vi "Perform Measurement.vi"(7 "error in (no error)":errorcluster, 8 "Measure Call Context in":refnum<class "Measure Call Context.lvclass">, 10 "measurement configuration":T2={"Mode of operation"=enum."Power on the DUT", "Source enable/disable"=FALSE, "Load enable/disable"=FALSE, "Source resource names"=[], "Load resource names"=[], "Power ON/Source system configuration"=enum."Series", "Power ON/Source output function"=0, "Source sweep scale"="", "Power ON V/I Source start level"=0.0, "Source stop level"=0.0, "Source sweep points/points per decade"=0, "Source voltage/current level range"=0.0, "Power ON/Source sense"=0, "Source limit symmetry"=enum."Symmetric", "Power ON/Source current/voltage limit range"=0.0, "Source current/voltage limit low"=0.0, "Source current/voltage limit high"=0.0, "Source source delay"=0.0, "Source aperture time"=0.0, "Source transient response"=0, "Source voltage/current gain bandwidth"=0.0, "Source voltage/current compensation frequency"=0.0, "Source voltage/current pole-zero ratio"=0.0, "Load system configuration"=enum."Series", "Load output function"=0, "Load device voltage/current rating"=50.0, "Load sweep scale"="", "Load start level"=0.0, "Load stop level"=0.0, "Load sweep points/points per decade"=0, "Load voltage/current level range"=0.0, "Load sense"=0, "Load limit symmetry"=enum."Symmetric", "Load current/voltage limit range"=0.0, "Load current/voltage limit low"=0.0, "Load current/voltage limit high"=0.0, "Load source delay"=0.0, "Load aperture time"=0.0, "Load transient response"=0, "Load voltage/current gain bandwidth"=0.0, "Load voltage/current compensation frequency"=0.0, "Load voltage/current pole-zero ratio"=0.0, "Load source trigger"="", "Load measure trigger"="", "Measurement timeout"=10.0} {"Measurement timeout" format="%.3p"; "Load device voltage/current rating" format="%#_6pA"; "Load output function" items=["DC Voltage"=1006, "DC Current"=1007, "Pulse Voltage"=1049, "Pulse Current"=1050]; "Power ON/Source output function" items=["DC Voltage"=1006, "DC Current"=1007, "Pulse Voltage"=1049, "Pulse Current"=1050]; "Load sweep points/points per decade" format="%#_6p"; "Power ON V/I Source start level" format="%#_6p"; "Load sense" items=["Symmetric", "Asymmetric"]; "Load transient response" items=["Slow"=1041, "Normal"=1038, "Fast"=1039, "Custom"=1042]; "Power ON/Source sense" items=["Local"=1008, "Remote"=1009]; "Source transient response" items=["Slow"=1041, "Normal"=1038, "Fast"=1039, "Custom"=1042]; "Load current/voltage limit low" format="%#_6p"; "Load current/voltage limit range" format="%#_6p"; "Load voltage/current level range" format="%#_6p"; "Source current/voltage limit high" format="%#_6p"; "Source current/voltage limit low" format="%#_6p"; "Power ON/Source current/voltage limit range" format="%#_6p"; "Source voltage/current level range" format="%#_6p"}) -> (0 "error out":errorcluster, 1 "Measure Call Context out":refnum<class "Measure Call Context.lvclass">, 3 "Measurement Results":T1)   [LabVIEW 2021, in "Sweep_Channel Ganging.lvlib"]
doc: "This VI Perform different API calls to do Sweep Measurement in different configurations of Source and Load like \n\nSingle-Ganged \nGanged-Ganged\nGanged-Single\nSingle-Single"
uses:
  Sweep_Channel Ganging.lvlib
  <vilib>/Plug-In SDKs/Measurements/Measure Call Context/Measure Call Context.lvclass
  Measurement Configuration.ctl
  Measurement Results.ctl
  Controls/Sweep perform meaasurement.ctl
  shared subVIs/ctl/NIDCPower_channel_ganging - ctl - ganged session.ctl
  shared subVIs/ctl/NIDCPower_channel_ganging - ctl - ganged config.ctl
  shared subVIs/ctl/NIDCPower_channel_ganging - ctl - channel mode.ctl
  shared/Single/controls/Initialize Resource Config-Single.ctl
  shared/Ganging/controls/Initialize Resource Config-Ganging.ctl
  shared/Single/controls/Source to Sequence Config-Single.ctl
  shared/Ganging/controls/Source to Sequence Config-Ganging.ctl
  shared/Single/controls/Load to Sequence Config-Single.ctl
  shared/Ganging/controls/Load to Sequence Config-Ganging.ctl
  <instrlib>/niDCPower/nidcpower.llb/niDCPower Wait For Event - Event.ctl
  shared/Common/controls/Start and Wait for Event.ctl
  Controls/Sweep fetch measurement control.ctl
  shared/Ganging/controls/Abort Single Point-Ganging.ctl
  shared/Single/controls/Abort Single Point-Single.ctl
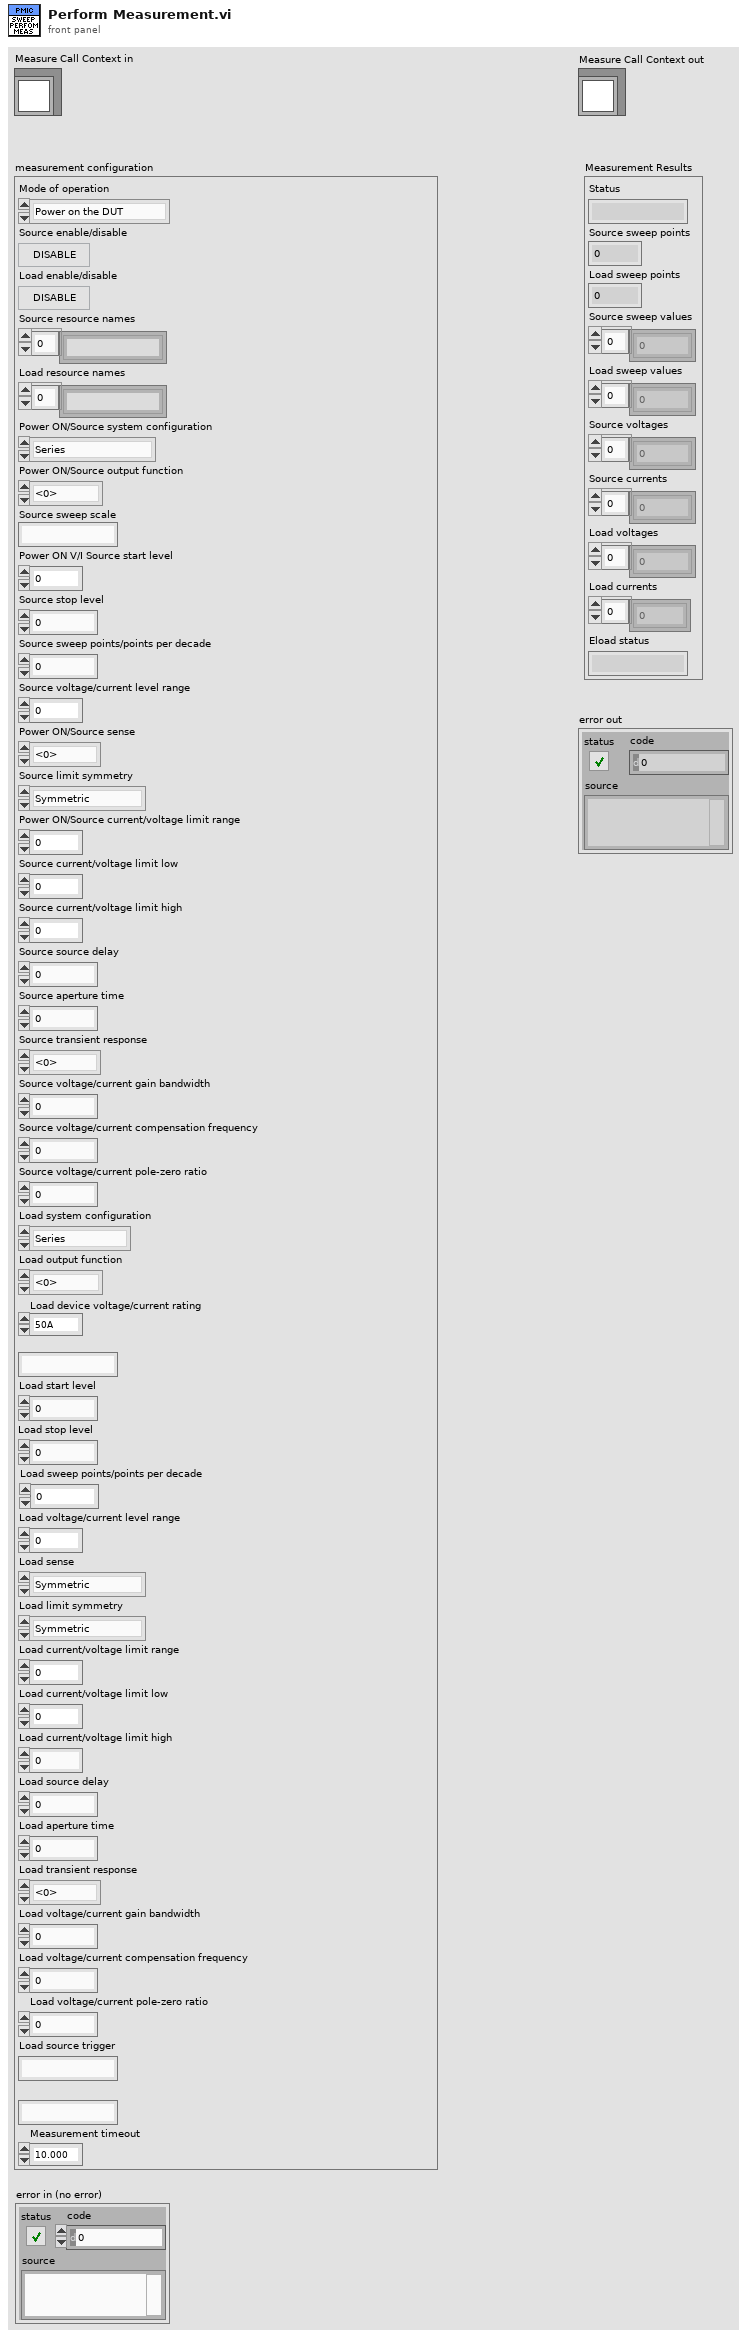
[diagram p1: front panel]
types:
  T1 = typedef "Sweep_Channel Ganging.lvlib/Measurement Results.ctl" = cluster{"Status":string, "Source sweep points":i32, "Load sweep points":i32, "Source sweep values":dbl[], "Load sweep values":dbl[], "Source voltages":dbl[], "Source currents":dbl[], "Load voltages":dbl[], "Load currents":dbl[], "Eload status":string}
  T2 = typedef "Sweep_Channel Ganging.lvlib/Measurement Configuration.ctl" = cluster{"Mode of operation":enum32{"Power on the DUT", "Perform measurement", "Power off the DUT"}, "Source enable/disable":bool, "Load enable/disable":bool, "Source resource names":string[], "Load resource names":string[], "Power ON/Source system configuration":enum32{"Series", "Parallel", "Manual"}, "Power ON/Source output function":i32, "Source sweep scale":string, "Power ON V/I Source start level":dbl, "Source stop level":dbl, "Source sweep points/points per decade":i32, "Source voltage/current level range":dbl, "Power ON/Source sense":i32, "Source limit symmetry":enum32{"Symmetric", "Asymmetric"}, "Power ON/Source current/voltage limit range":dbl, "Source current/voltage limit low":dbl, "Source current/voltage limit high":dbl, "Source source delay":dbl, "Source aperture time":dbl, "Source transient response":i32, "Source voltage/current gain bandwidth":dbl, "Source voltage/current compensation frequency":dbl, "Source voltage/current pole-zero ratio":dbl, "Load system configuration":enum32{"Series", "Parallel", "Manual"}, "Load output function":i32, "Load device voltage/current rating":dbl, "Load sweep scale":string, "Load start level":dbl, "Load stop level":dbl, "Load sweep points/points per decade":i32, "Load voltage/current level range":dbl, "Load sense":i32, "Load limit symmetry":enum32{"Symmetric", "Asymmetric"}, "Load current/voltage limit range":dbl, "Load current/voltage limit low":dbl, "Load current/voltage limit high":dbl, "Load source delay":dbl, "Load aperture time":dbl, "Load transient response":i32, "Load voltage/current gain bandwidth":dbl, "Load voltage/current compensation frequency":dbl, "Load voltage/current pole-zero ratio":dbl, "Load source trigger":string, "Load measure trigger":string, "Measurement timeout":dbl}
  T3 = typedef "Sweep_Channel Ganging.lvlib/Sweep perform meaasurement.ctl" = cluster{"Source Ganged Session Out":T4, "Load Ganged Session Out":T4, "Source sweep values":dbl[], "Source sweep points":i32, "Load sweep values":dbl[], "Load sweep points":i32, "Measurement Results":T1, "Source Master/Single resource name":string, "Source Slave resource name":string[], "Load Master/Single resource name":string, "Load Slave resource name":string[], "Load ganged/single":bool, "Source ganged/single":bool, "Source channel name":string, "Load channel name":string, "Source session out":refnum<k15>, "Load session out":refnum<k15>, "Number of Eload used":i32, "Load Source ON/OFF":enum16{"SOURCE AND LOAD OFF", "SOURCE ON", "LOAD ON", "SOURCE AND LOAD ON"}}
  T4 = typedef "NIDCPower_channel_ganging - ctl - ganged session.ctl" = cluster{"Ganged Config":T5, "Session List":refnum<k15>[], "Session Mode":T6[], "Channel":string[]}
  T5 = typedef "NIDCPower_channel_ganging - ctl - ganged config.ctl" = enum32{"Series", "Parallel", "Manual"}
  T6 = typedef "NIDCPower_channel_ganging - ctl - channel mode.ctl" = enum32{"Master", "Slave", "Slave - Inverted"}
  T7 = typedef "Initialize Resource Config-Single.ctl" = cluster{"Resource name":string, "Voltage/current level":dbl, "Voltage/current level range":dbl, "Voltage/current limit range":dbl, "Voltage/current limit low":dbl, "Voltage/current limit high":dbl, "Output function":i32, "Sense":i32, "Transient response":i32, "Voltage/current gain bandwidth":dbl, "Voltage/current compensation frequency":dbl, "Voltage/current pole-zero ratio":dbl, "DUT set-up time":dbl, "Limit symmetry":enum32{"Symmetric", "Asymmetric"}}
  T8 = typedef "Initialize Resource Config-Ganging.ctl" = cluster{"Master resource name ":string, "Slave resource names":string[], "System configuration":enum32{"Series", "Parallel", "Manual"}, "Voltage/current level":dbl, "Voltage/current level range":dbl, "Limit symmetry":enum32{"Symmetric", "Asymmetric"}, "Voltage/current limit range":dbl, "Voltage/current limit low":dbl, "Voltage/current limit high":dbl, "Output function":i32, "Sense":i32, "Transient response":i32, "Voltage/current gain bandwith":dbl, "Voltage/current compensation frequency":dbl, "Voltage/current pole-zero ratio":dbl, "DUT set-up time":dbl}
  T9 = typedef "Source to Sequence Config-Single.ctl" = cluster{"Source channel name":string, "Source out":refnum<k15>, "Source sweep values":dbl[], "Load sweep points":i32, "Source output function":i32, "Source transient response":i32, "Source voltage/current gain bandwidth":dbl, "Source voltage/current compensation frequency":dbl, "Source voltage/current pole-zero ratio":dbl, "Source aperture time":dbl, "Source source delay":dbl}
  T10 = typedef "Source to Sequence Config-Ganging.ctl" = cluster{"Source Ganged Session Out":cluster{"Ganged Config":T5, "Session List":refnum<k15>[], "Session Mode":T6[], "Channel":string[]}, "Source sweep values":dbl[], "Load sweep points":i32, "Source output function":i32, "Source transient response":i32, "Source voltage/current gain bandwidth":dbl, "Source voltage/current compensation frequency":dbl, "Source voltage/current pole-zero ratio":dbl, "Source aperture time":dbl, "Source source delay":dbl}
  T11 = typedef "Load to Sequence Config-Single.ctl" = cluster{"Load channel name":string, "Load out":refnum<k15>, "Load sweep values":dbl[], "Source sweep points":i32, "Load output function":i32, "Load transient response":i32, "Load voltage/current gain bandwidth":dbl, "Load voltage/current compensation frequency":dbl, "Load voltage/current pole-zero ratio":dbl, "Load aperture time":dbl, "Load source delay":dbl, "Load measure trigger":string, "Load source trigger":string}
  T12 = typedef "Load to Sequence Config-Ganging.ctl" = cluster{"Load Ganged Session Out":cluster{"Ganged Config":T5, "Session List":refnum<k15>[], "Session Mode":T6[], "Channel":string[]}, "Load sweep values":dbl[], "Source sweep points":i32, "Load output function":i32, "Load transient response":i32, "Load voltage/current gain bandwidth":dbl, "Load voltage/current compensation frequency":dbl, "Load voltage/current pole-zero ratio":dbl, "Load aperture time":dbl, "Load source delay":dbl, "Load measure trigger":string, "Load source trigger":string}
  T13 = typedef "Start and Wait for Event.ctl" = cluster{"Source Ganged Session Out":T4, "Load Ganged Session Out":T4, "Source session out":refnum<k15>, "Load session out":refnum<k15>, "event":T14, "Source channel name":string, "Load channel name":string, "Load Source ON/OFF":enum16{"SOURCE AND LOAD OFF", "SOURCE ON", "LOAD ON", "SOURCE AND LOAD ON"}, "Load ganged/single":bool, "Source ganged/single":bool}
  T14 = typedef "niDCPower Wait For Event - Event.ctl" = i32
  T15 = typedef "Sweep_Channel Ganging.lvlib/Sweep fetch measurement control.ctl" = cluster{"Source Ganged Session Out":T4, "Load Ganged Session Out":T4, "Source sweep values":dbl[], "Source sweep points":i32, "Load sweep values":dbl[], "Load sweep points":i32, "Measurement Results":T1, "Load ganged/single":bool, "Source ganged/single":bool, "Source channel name":string, "Load channel name":string, "Source session out":refnum<k15>, "Load session out":refnum<k15>, "Load Source ON/OFF":enum16{"SOURCE AND LOAD OFF", "SOURCE ON", "LOAD ON", "SOURCE AND LOAD ON"}, "Measurement timeout":dbl}
  T16 = typedef "Abort Single Point-Ganging.ctl" = cluster{"Ganged Session in":cluster{"Ganged Config":T5, "Session List":refnum<k15>[], "Session Mode":T6[], "Channel":string[]}}
  T17 = typedef "Abort Single Point-Single.ctl" = cluster{"Resource out":refnum<k15>, "Resource channel name":string}
  T18 = enum32{"Power on the DUT", "Perform measurement", "Power off the DUT"}
  T19 = enum16{"SOURCE AND LOAD OFF", "SOURCE ON", "LOAD ON", "SOURCE AND LOAD ON"}
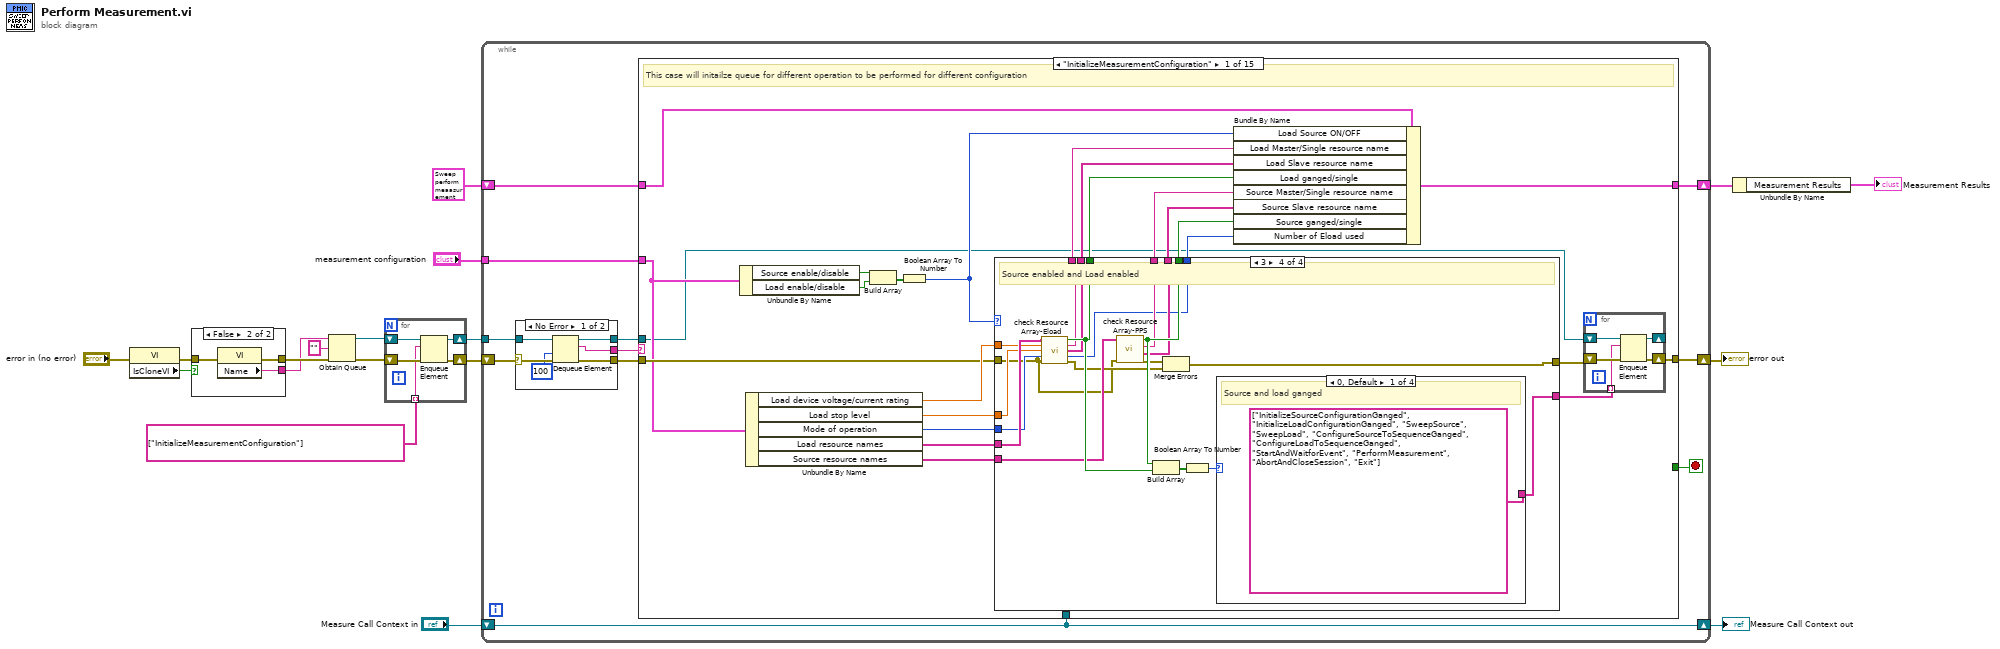
[diagram p0: block diagram]
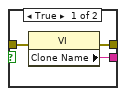
[diagram p2: hidden frame]
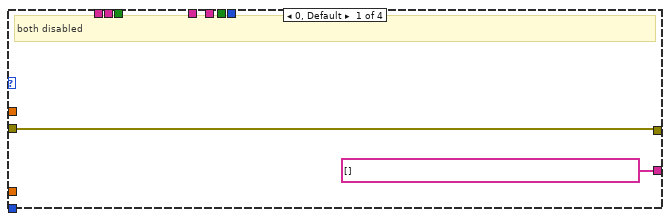
[diagram p3: hidden frame]
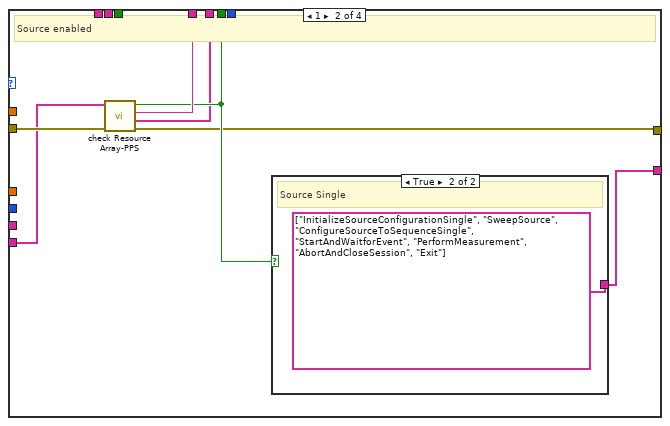
[diagram p4: hidden frame]
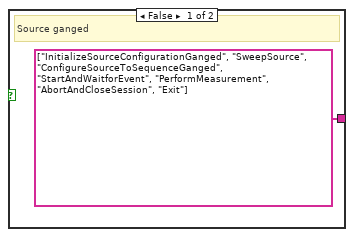
[diagram p5: hidden frame]
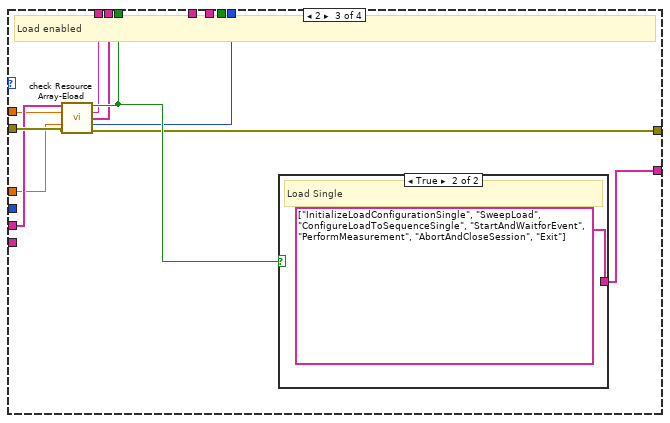
[diagram p6: hidden frame]
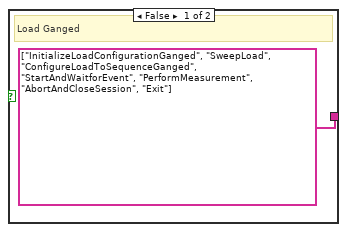
[diagram p7: hidden frame]
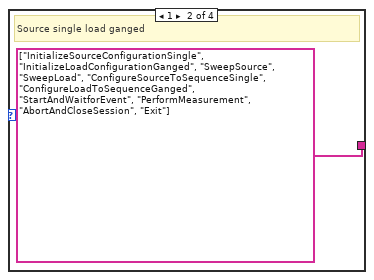
[diagram p8: hidden frame]
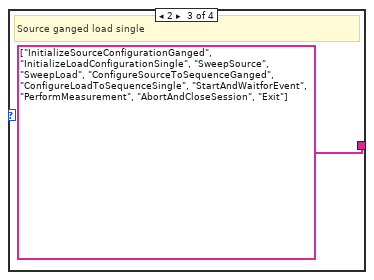
[diagram p9: hidden frame]
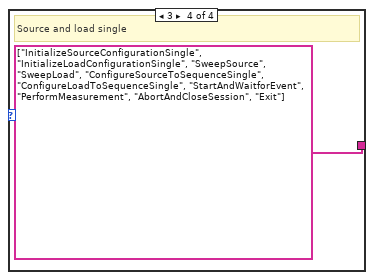
[diagram p10: hidden frame]
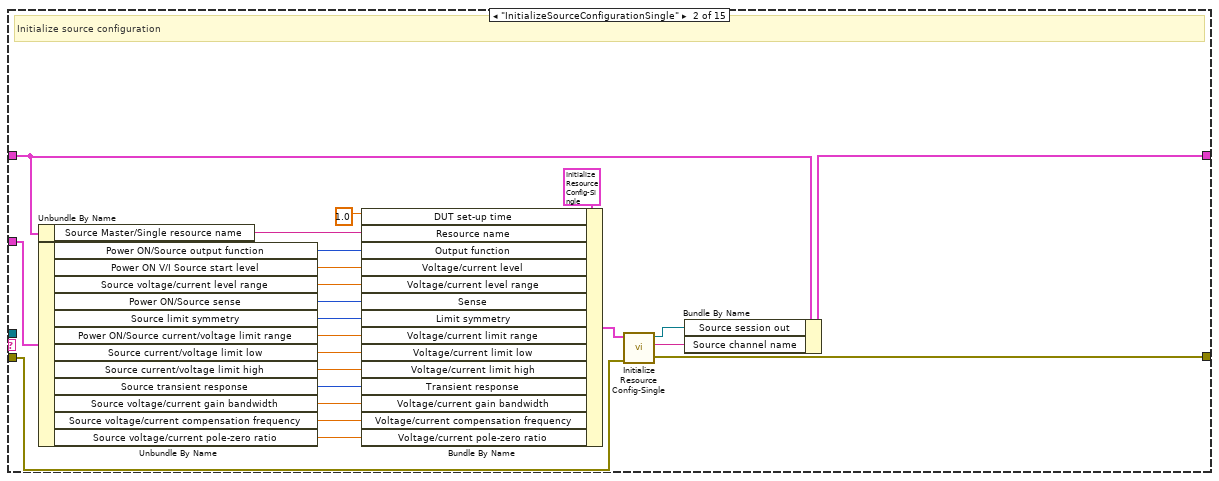
[diagram p11: hidden frame]
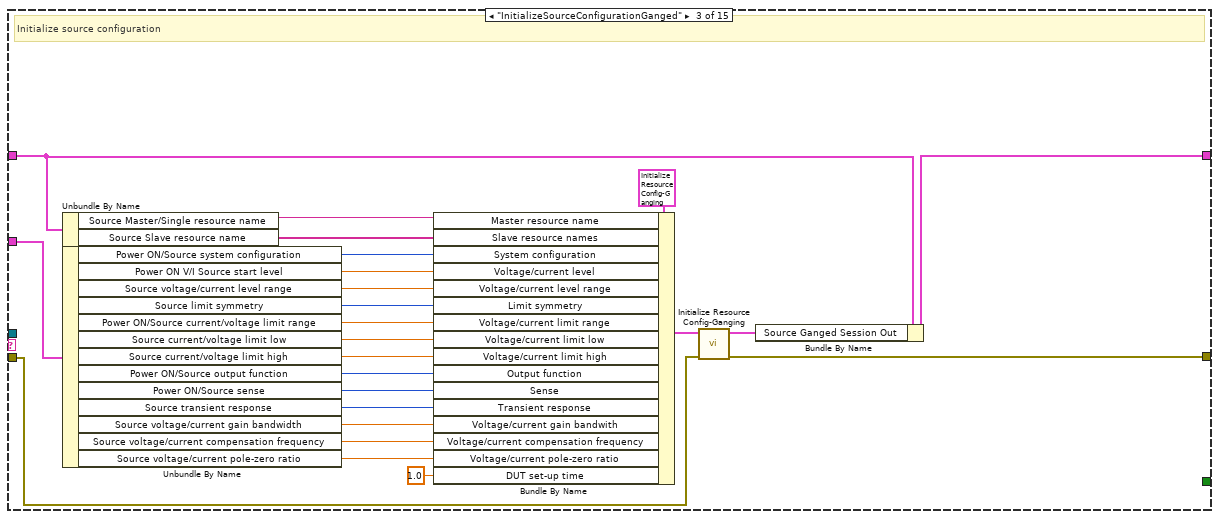
[diagram p12: hidden frame]
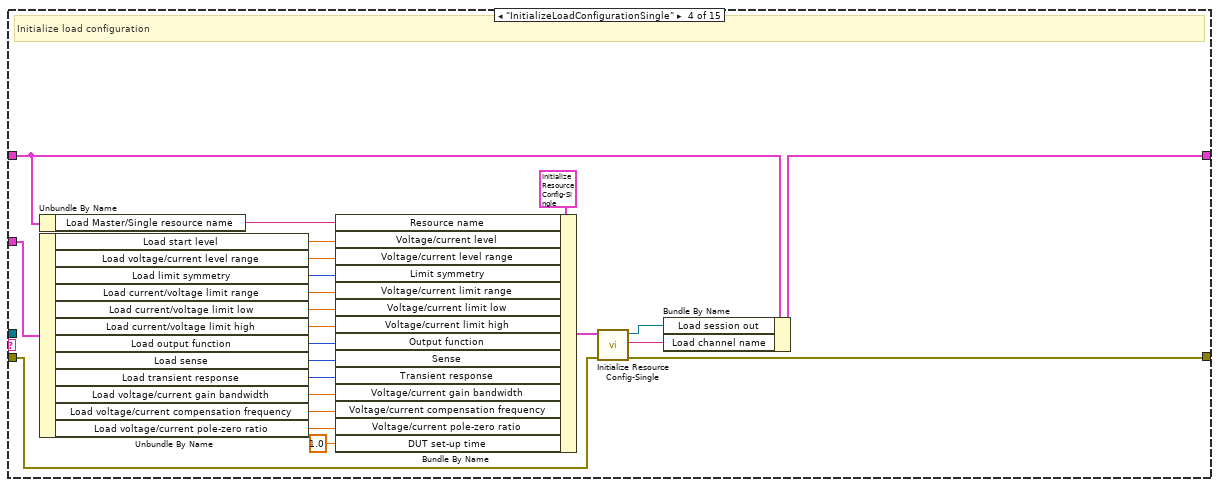
[diagram p13: hidden frame]
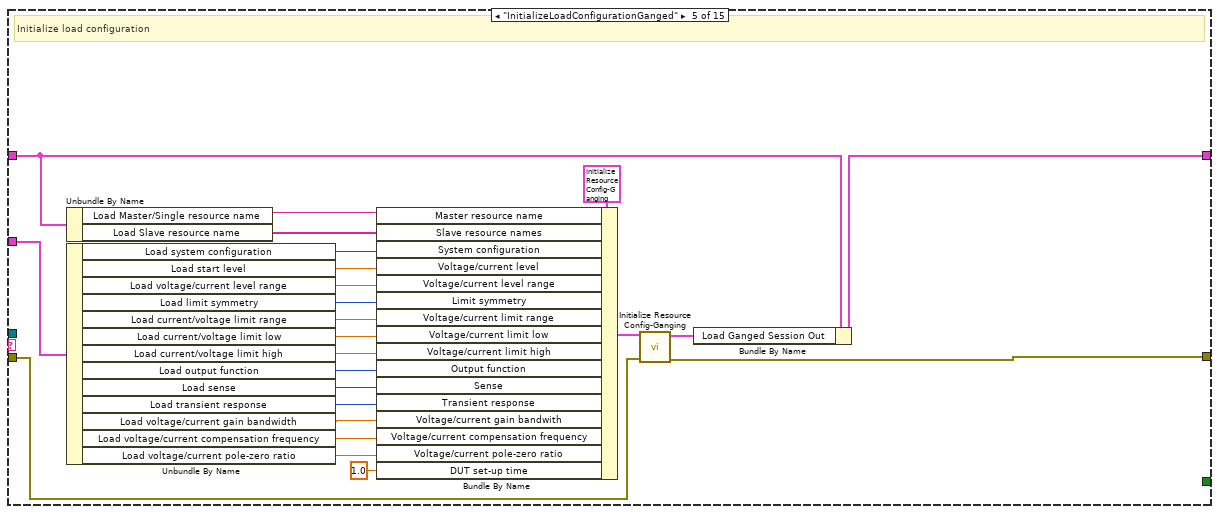
[diagram p14: hidden frame]
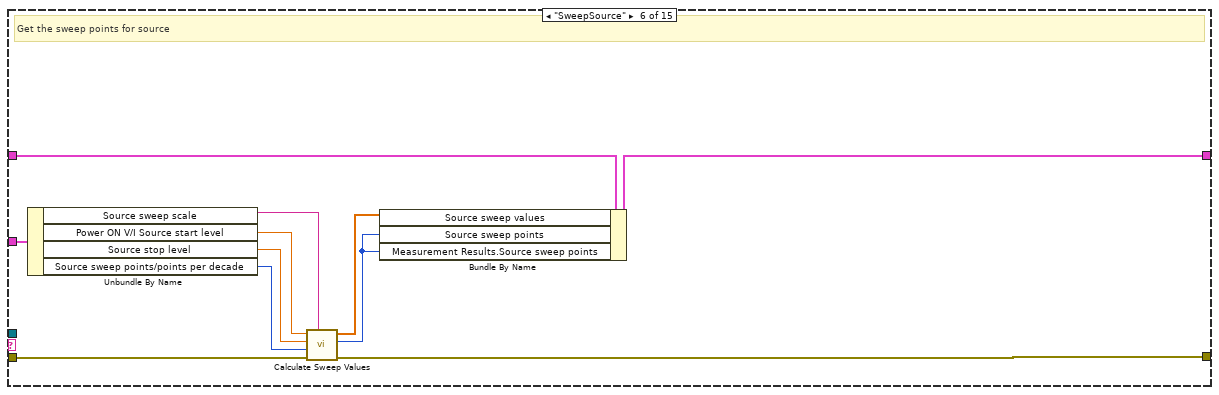
[diagram p15: hidden frame]
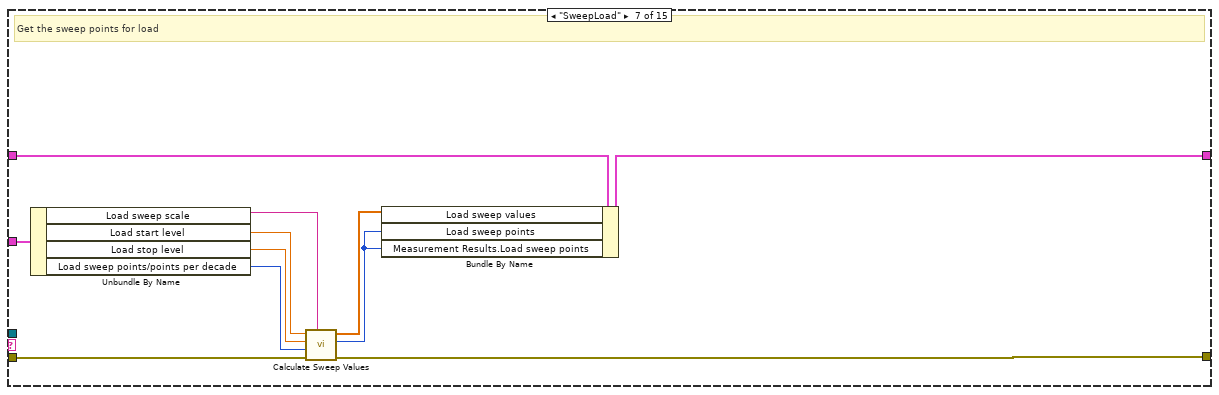
[diagram p16: hidden frame]
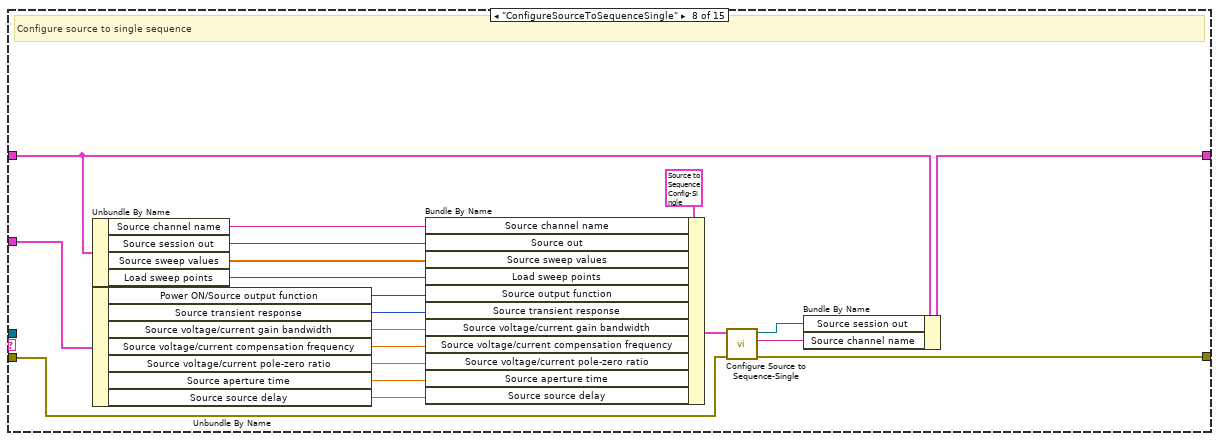
[diagram p17: hidden frame]
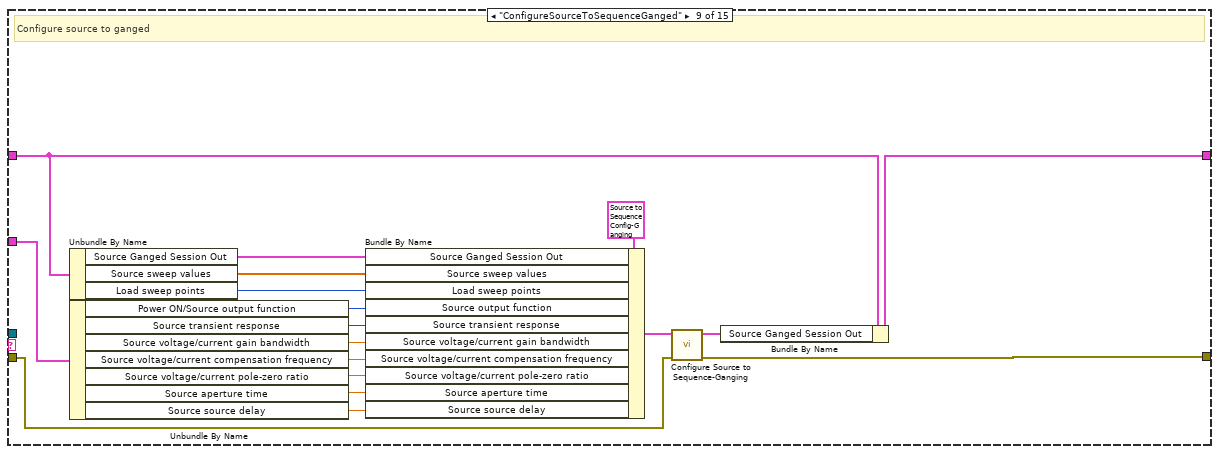
[diagram p18: hidden frame]
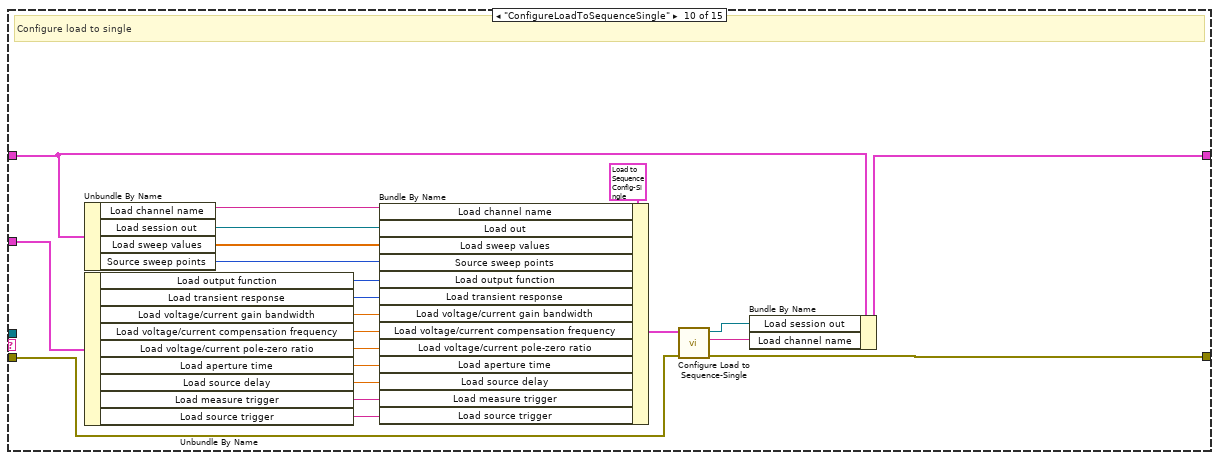
[diagram p19: hidden frame]
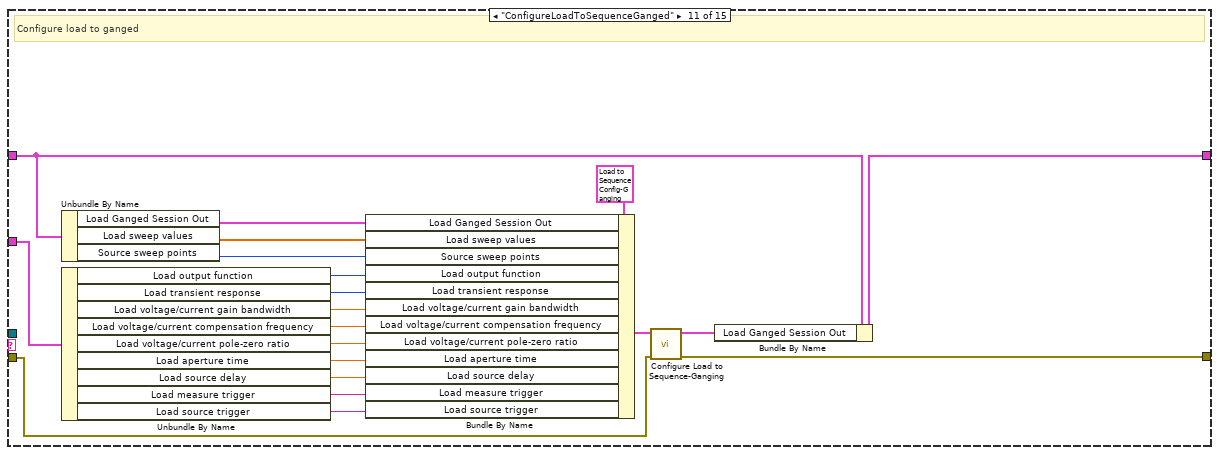
[diagram p20: hidden frame]
diagram:
  n1 = property class="VI"(error in="error in (no error)") -> (error out=w14:errorcluster, "IsCloneVI"=w13:bool)  [unwired: 1 in, 1 out]
  n2 = case shown="False" w13 {
    tunnel: [w21 w24] -> w6
    tunnel: [w20 w23] -> w4
    tunnel: w14 -> [w19 w22]
    frame True {
      n3 = property class="VI"(error in=w19) -> (error out=w21:errorcluster, "Clone Name"=w20:string)  [unwired: 1 in, 1 out]
    }
    frame False {
      n4 = property class="VI"(error in=w22) -> (error out=w24:errorcluster, "Name"=w23:string)  [unwired: 1 in, 1 out]
    }
  }
  n5 = Obtain Queue(name (unnamed)=w4, element data type="", error in (no error)=w6) -> (queue out=w9:refnum<queue>, error out=w10:errorcluster)  [unwired: 2 in, 1 out]
  n6 = for {
    shift-right: [w28] -> w5
    shift-left: w9 -> [w26]
    shift-right: [w27] -> w7
    shift-left: w10 -> [w29]
    tunnel: string[] ["InitializeMeasurementConfiguration"] ("Step sequence") -> [w25] mode=indexing
    n7 = Enqueue Element(queue=w26, element=w25, error in (no error)=w29) -> (queue out=w28:refnum<queue>, error out=w27:errorcluster)  [unwired: 1 in, 1 out]
  }
  n8 = while {
    shift-right: [w35] -> w2
    shift-left: T3 {"Source Ganged Session Out"={"Ganged Config"=enum."Series", "Session List"=[], "Session Mode"=[], "Channel"=[]}, "Load Ganged Session Out"={"Ganged Config"=enum."Series", "Session List"=[], "Session Mode"=[], "Channel"=[]}, "Source sweep values"=[], "Source sweep points"=0, "Load sweep values"=[], "Load sweep points"=0, "Measurement Results"={"Status"="", "Source sweep points"=0, "Load sweep points"=0, "Source sweep values"=[], "Load sweep values"=[], "Source voltages"=[], "Source currents"=[], "Load voltages"=[], "Load currents"=[], "Eload status"=""}, "Source Master/Single resource name"="", "Source Slave resource name"=[], "Load Master/Single resource name"="", "Load Slave resource name"=[], "Load ganged/single"=FALSE, "Source ganged/single"=FALSE, "Source channel name"="", "Load channel name"="", "Source session out"="", "Load session out"="", "Number of Eload used"=0, "Load Source ON/OFF"=enum."SOURCE AND LOAD OFF"} ("Sweep perform measurement control") -> [w36]
    shift-right: [w31] -> w17
    shift-left: w7 -> [w40]
    shift-right: [w34] -> w15
    shift-left: "Measure Call Context in" -> [w34]
    tunnel: "measurement configuration" -> [w32]
    tunnel: w5 -> [w30]
    stop <- w33 stop-if-true
    n9 = case shown="No Error" w40 {
      selector: w40 -> [w484 w487]
      tunnel: [w485 "Exit" ("t")] -> w39
      tunnel: [w483 w487] -> w37
      tunnel: [w481 w486] -> w38
      tunnel: w30 -> [w480 w486]
      frame No Error {
        n10 = Dequeue Element(queue=w480, timeout in ms (-1)=100, error in (no error)=w484) -> (queue out=w481:refnum<queue>, element=w485:string, error out=w483:errorcluster)  [unwired: 1 out]
      }
      frame Error {
      }
    }
    n11 = case shown="\"InitializeMeasurementConfiguration\"" w39 {
      tunnel: w38 -> [w42 _ _ _ _ _ _ _ _ _ _ _ _ _ w471]
      tunnel: w37 -> [w48 w118 w144 w165 w205 w220 w231 w235 w255 w274 w295 w317 w340 w360 w473]
      tunnel: w36 -> [w49 w122 w142 w167 w204 w214 w225 w248 w266 w289 w309 w325 w355 w362 w475]
      tunnel: [w50 w121 w143 w166 w203 w211 w224 w249 w269 w291 w311 w324 w357 w364 w475] -> w35
      tunnel: w34 -> [_ _ _ _ _ _ _ _ _ _ _ _ w338 _ _]
      tunnel: [_ _ _ _ _ _ _ _ _ _ _ _ _ TRUE TRUE] -> w33
      tunnel: w32 -> [w47 w138 w145 w183 w206 w219 w230 w247 w267 w288 w308 _ w336 _ _]
      tunnel: [w45 w117 w140 w164 w187 w210 w222 w234 w254 w273 w294 w316 w359 w363 w472] -> w31
      frame "InitializeMeasurementConfiguration" {
        # "This case will initailze queue for different operation to be performed for different configuration"
        n12 = Unbundle By Name(w47) -> ("Source enable/disable"=w53:bool, "Load enable/disable"=w52:bool)
        n13 = Unbundle By Name(w47) -> ("Load device voltage/current rating"=w63:dbl, "Load stop level"=w64:dbl, "Mode of operation"=w41:T18, "Load resource names"=w54:string[], "Source resource names"=w55:string[])
        n14 = Build Array(w53, w52) -> (w51:bool[])
        n15 = Boolean Array To Number(Boolean array=w51) -> (number=w56:u32)
        n16 = case shown="3" w56 {
          tunnel: w48 -> [w70 w78 w90 w93]
          tunnel: [w70 w73 w83 w95] -> w44
          tunnel: w54 -> [_ _ w89 w109]
          tunnel: w55 -> [_ w77 _ w102]
          tunnel: [_ _ w87 w107] -> w57
          tunnel: [_ _ w86 w106] -> w58
          tunnel: [_ w76 _ w104] -> w59
          tunnel: [_ w74 _ w103] -> w60
          tunnel: [_ _ w88 w108] -> w61
          tunnel: [_ w75 _ w105] -> w62
          tunnel: w63 -> [_ _ w85 w101]
          tunnel: w64 -> [_ _ w84 w97]
          tunnel: [string[] [] ("Step sequence") w72 w82 w98] -> w46
          tunnel: [_ _ w81 w99] -> w43
          tunnel: w41 -> [_ _ _ w96]
          frame 0, Default {
            # "both disabled"
          }
          frame 1 {
            # "Source enabled"
            n17 = call "check Resource Array-PPS.vi"("error in"=w78, "Resource names"=w77) -> ("error out"=w73:errorcluster, "Slave resource names"=w74:string[], "Single/Master resouce names"=w76:string, "Single or ganged configuration"=w75:bool)  [unwired: 6 in]
            n18 = case shown="True" w75 {
              tunnel: [string[] ["InitializeSourceConfigurationGanged", "SweepSource", "ConfigureSourceToSequenceGanged", "StartAndWaitforEvent", "PerformMeasurement", "AbortAndCloseSession", "Exit"] ("Step sequence") string[] ["InitializeSourceConfigurationSingle", "SweepSource", "ConfigureSourceToSequenceSingle", "StartAndWaitforEvent", "PerformMeasurement", "AbortAndCloseSession", "Exit"] ("Step sequence")] -> w72
              frame False {
                # "Source ganged"
              }
              frame True {
                # "Source Single"
              }
            }
          }
          frame 2 {
            # "Load enabled"
            n19 = call "check Resource Array-Eload.vi"("Resource names"=w89, "Device current rating"=w85, "Mode of operation"=w84, "error in"=w90) -> ("Single or ganged configuration"=w88:bool, "Single/Master resouce name"=w87:string, "Slave resource names"=w86:string[], "Number of devices used"=w81:i32, "error out"=w83:errorcluster)  [unwired: 7 in]
            n20 = case shown="True" w88 {
              tunnel: [string[] ["InitializeLoadConfigurationGanged", "SweepLoad", "ConfigureLoadToSequenceGanged", "StartAndWaitforEvent", "PerformMeasurement", "AbortAndCloseSession", "Exit"] ("Step sequence") string[] ["InitializeLoadConfigurationSingle", "SweepLoad", "ConfigureLoadToSequenceSingle", "StartAndWaitforEvent", "PerformMeasurement", "AbortAndCloseSession", "Exit"] ("Step sequence")] -> w82
              frame False {
                # "Load Ganged"
              }
              frame True {
                # "Load Single"
              }
            }
          }
          frame 3 {
            # "Source enabled and Load enabled"
            n21 = call "check Resource Array-Eload.vi"("Resource names"=w109, "Device current rating"=w101, "Expected current level"=w97, "Mode of operation"=w96, "error in"=w93) -> ("Single or ganged configuration"=w108:bool, "Single/Master resouce name"=w107:string, "Slave resource names"=w106:string[], "Number of devices used"=w99:i32, "error out"=w94:errorcluster)  [unwired: 6 in]
            n22 = call "check Resource Array-PPS.vi"("error in"=w93, "Resource names"=w102) -> ("error out"=w100:errorcluster, "Slave resource names"=w103:string[], "Single/Master resouce names"=w104:string, "Single or ganged configuration"=w105:bool)  [unwired: 6 in]
            n23 = Build Array(w105, w108) -> (w111:bool[])
            n24 = Merge Errors(w100, w94) -> (w95:errorcluster)
            n25 = Boolean Array To Number(Boolean array=w111) -> (number=w110:u32)
            n26 = case shown="0, Default" w110 {
              tunnel: [string[] ["InitializeSourceConfigurationGanged", "InitializeLoadConfigurationGanged", "SweepSource", "SweepLoad", "ConfigureSourceToSequenceGanged", "ConfigureLoadToSequenceGanged", "StartAndWaitforEvent", "PerformMeasurement", "AbortAndCloseSession", "Exit"] ("Step sequence") string[] ["InitializeSourceConfigurationSingle", "InitializeLoadConfigurationGanged", "SweepSource", "SweepLoad", "ConfigureSourceToSequenceSingle", "ConfigureLoadToSequenceGanged", "StartAndWaitforEvent", "PerformMeasurement", "AbortAndCloseSession", "Exit"] ("Step sequence") string[] ["InitializeSourceConfigurationGanged", "InitializeLoadConfigurationSingle", "SweepSource", "SweepLoad", "ConfigureSourceToSequenceGanged", "ConfigureLoadToSequenceSingle", "StartAndWaitforEvent", "PerformMeasurement", "AbortAndCloseSession", "Exit"] ("Step sequence") string[] ["InitializeSourceConfigurationSingle", "InitializeLoadConfigurationSingle", "SweepSource", "SweepLoad", "ConfigureSourceToSequenceSingle", "ConfigureLoadToSequenceSingle", "StartAndWaitforEvent", "PerformMeasurement", "AbortAndCloseSession", "Exit"] ("Step sequence")] -> w98
              frame 0, Default {
                # "Source and load ganged"
              }
              frame 1 {
                # "Source single load ganged"
              }
              frame 2 {
                # "Source ganged load single"
              }
              frame 3 {
                # "Source and load single"
              }
            }
          }
        }
        n27 = Bundle By Name(cluster=w49, "Load Source ON/OFF"=w56, "Load Master/Single resource name"=w57, "Load Slave resource name"=w58, "Load ganged/single"=w61, "Source Master/Single resource name"=w59, "Source Slave resource name"=w60, "Source ganged/single"=w62, "Number of Eload used"=w43) -> (w50:T3)
        n28 = for {
          shift-right: [w67] -> _
          shift-left: w42 -> [w69]
          shift-right: [w66] -> w45
          shift-left: w44 -> [w68]
          tunnel: w46 -> [w65] mode=indexing
          n29 = Enqueue Element(queue=w69, element=w65, error in (no error)=w68) -> (queue out=w67:refnum<queue>, error out=w66:errorcluster)  [unwired: 1 in, 1 out]
        }
      }
      frame "InitializeSourceConfigurationSingle" {
        # "Initialize source configuration"
        n30 = Unbundle By Name(w122) -> ("Source Master/Single resource name"=w123:string)
        n31 = Unbundle By Name(w138) -> ("Power ON/Source output function"=w137:i32, "Power ON V/I Source start level"=w136:dbl, "Source voltage/current level range"=w135:dbl, "Power ON/Source sense"=w134:i32, "Source limit symmetry"=w133:enum32{"Symmetric", "Asymmetric"}, "Power ON/Source current/voltage limit range"=w132:dbl, "Source current/voltage limit low"=w131:dbl, "Source current/voltage limit high"=w130:dbl, "Source transient response"=w129:i32, "Source voltage/current gain bandwidth"=w128:dbl, "Source voltage/current compensation frequency"=w127:dbl, "Source voltage/current pole-zero ratio"=w126:dbl)
        n32 = Bundle By Name(cluster=T7 {"Resource name"="", "Voltage/current level"=0.0, "Voltage/current level range"=0.0, "Voltage/current limit range"=0.0, "Voltage/current limit low"=0.0, "Voltage/current limit high"=inf, "Output function"=1007, "Sense"=1009, "Transient response"=1038, "Voltage/current gain bandwidth"=0.0, "Voltage/current compensation frequency"=0.0, "Voltage/current pole-zero ratio"=0.0, "DUT set-up time"=0.0, "Limit symmetry"=enum."Symmetric"} ("Initialize Resource Config - Single"), "DUT set-up time"=1.0, "Resource name"=w123, "Output function"=w137, "Voltage/current level"=w136, "Voltage/current level range"=w135, "Sense"=w134, "Limit symmetry"=w133, "Voltage/current limit range"=w132, "Voltage/current limit low"=w131, "Voltage/current limit high"=w130, "Transient response"=w129, "Voltage/current gain bandwidth"=w128, "Voltage/current compensation frequency"=w127, "Voltage/current pole-zero ratio"=w126) -> (w124:T7)
        n33 = call "Initialize Resource Config-Single.vi"("error in"=w118, "Initialize resource Config - Single"=w124) -> ("error out"=w117:errorcluster, "channel name"=w120:string, "instrument handle out"=w119:refnum<k15>)  [unwired: 7 in]
        n34 = Bundle By Name(cluster=w122, "Source session out"=w119, "Source channel name"=w120) -> (w121:T3)
      }
      frame "InitializeSourceConfigurationGanged" {
        # "Initialize source configuration"
        n35 = Unbundle By Name(w142) -> ("Source Master/Single resource name"=w160:string, "Source Slave resource name"=w159:string[])
        n36 = Unbundle By Name(w145) -> ("Power ON/Source system configuration"=w158:enum32{"Series", "Parallel", "Manual"}, "Power ON V/I Source start level"=w157:dbl, "Source voltage/current level range"=w156:dbl, "Source limit symmetry"=w155:enum32{"Symmetric", "Asymmetric"}, "Power ON/Source current/voltage limit range"=w146:dbl, "Source current/voltage limit low"=w147:dbl, "Source current/voltage limit high"=w148:dbl, "Power ON/Source output function"=w149:i32, "Power ON/Source sense"=w150:i32, "Source transient response"=w151:i32, "Source voltage/current gain bandwidth"=w154:dbl, "Source voltage/current compensation frequency"=w153:dbl, "Source voltage/current pole-zero ratio"=w152:dbl)
        n37 = Bundle By Name(cluster=T8 {"Master resource name "="", "Slave resource names"=[], "System configuration"=enum."Parallel", "Voltage/current level"=0.0, "Voltage/current level range"=0.0, "Limit symmetry"=enum."Symmetric", "Voltage/current limit range"=0.0, "Voltage/current limit low"=0.0, "Voltage/current limit high"=inf, "Output function"=1007, "Sense"=1009, "Transient response"=1038, "Voltage/current gain bandwith"=0.0, "Voltage/current compensation frequency"=0.0, "Voltage/current pole-zero ratio"=0.0, "DUT set-up time"=0.0} ("Initialize Resource Config - Ganging"), "Master resource name"=w160, "Slave resource names"=w159, "System configuration"=w158, "Voltage/current level"=w157, "Voltage/current level range"=w156, "Limit symmetry"=w155, "Voltage/current limit range"=w146, "Voltage/current limit low"=w147, "Voltage/current limit high"=w148, "Output function"=w149, "Sense"=w150, "Transient response"=w151, "Voltage/current gain bandwith"=w154, "Voltage/current compensation frequency"=w153, "Voltage/current pole-zero ratio"=w152, "DUT set-up time"=1.0) -> (w162:T8)
        n38 = call "Initialize Resource Config-Ganging.vi"("error in"=w144, "Initialize Resource Config - Ganging"=w162) -> ("error out"=w140:errorcluster, "Ganged Session Out"=w141:T4)  [unwired: 8 in]
        n39 = Bundle By Name(cluster=w142, "Source Ganged Session Out"=w141) -> (w143:T3)
      }
      frame "InitializeLoadConfigurationSingle" {
        # "Initialize load configuration"
        n40 = Unbundle By Name(w167) -> ("Load Master/Single resource name"=w182:string)
        n41 = Unbundle By Name(w183) -> ("Load start level"=w170:dbl, "Load voltage/current level range"=w171:dbl, "Load limit symmetry"=w172:enum32{"Symmetric", "Asymmetric"}, "Load current/voltage limit range"=w173:dbl, "Load current/voltage limit low"=w174:dbl, "Load current/voltage limit high"=w175:dbl, "Load output function"=w176:i32, "Load sense"=w177:i32, "Load transient response"=w181:i32, "Load voltage/current gain bandwidth"=w180:dbl, "Load voltage/current compensation frequency"=w179:dbl, "Load voltage/current pole-zero ratio"=w178:dbl)
        n42 = Bundle By Name(cluster=T7 {"Resource name"="", "Voltage/current level"=0.0, "Voltage/current level range"=0.0, "Voltage/current limit range"=0.0, "Voltage/current limit low"=0.0, "Voltage/current limit high"=inf, "Output function"=1007, "Sense"=1009, "Transient response"=1038, "Voltage/current gain bandwidth"=0.0, "Voltage/current compensation frequency"=0.0, "Voltage/current pole-zero ratio"=0.0, "DUT set-up time"=0.0, "Limit symmetry"=enum."Symmetric"} ("Initialize Resource Config - Single"), "Resource name"=w182, "Voltage/current level"=w170, "Voltage/current level range"=w171, "Limit symmetry"=w172, "Voltage/current limit range"=w173, "Voltage/current limit low"=w174, "Voltage/current limit high"=w175, "Output function"=w176, "Sense"=w177, "Transient response"=w181, "Voltage/current gain bandwidth"=w180, "Voltage/current compensation frequency"=w179, "Voltage/current pole-zero ratio"=w178, "DUT set-up time"=1.0) -> (w184:T7)
        n43 = call "Initialize Resource Config-Single.vi"("error in"=w165, "Initialize resource Config - Single"=w184) -> ("error out"=w164:errorcluster, "channel name"=w168:string, "instrument handle out"=w169:refnum<k15>)  [unwired: 7 in]
        n44 = Bundle By Name(cluster=w167, "Load session out"=w169, "Load channel name"=w168) -> (w166:T3)
      }
      frame "InitializeLoadConfigurationGanged" {
        # "Initialize load configuration"
        n45 = Unbundle By Name(w204) -> ("Load Master/Single resource name"=w202:string, "Load Slave resource name"=w201:string[])
        n46 = Unbundle By Name(w206) -> ("Load system configuration"=w200:enum32{"Series", "Parallel", "Manual"}, "Load start level"=w199:dbl, "Load voltage/current level range"=w198:dbl, "Load limit symmetry"=w197:enum32{"Symmetric", "Asymmetric"}, "Load current/voltage limit range"=w196:dbl, "Load current/voltage limit low"=w195:dbl, "Load current/voltage limit high"=w194:dbl, "Load output function"=w193:i32, "Load sense"=w192:i32, "Load transient response"=w191:i32, "Load voltage/current gain bandwidth"=w190:dbl, "Load voltage/current compensation frequency"=w189:dbl, "Load voltage/current pole-zero ratio"=w188:dbl)
        n47 = Bundle By Name(cluster=T8 {"Master resource name "="", "Slave resource names"=[], "System configuration"=enum."Parallel", "Voltage/current level"=0.0, "Voltage/current level range"=0.0, "Limit symmetry"=enum."Symmetric", "Voltage/current limit range"=0.0, "Voltage/current limit low"=0.0, "Voltage/current limit high"=inf, "Output function"=1007, "Sense"=1009, "Transient response"=1038, "Voltage/current gain bandwith"=0.0, "Voltage/current compensation frequency"=0.0, "Voltage/current pole-zero ratio"=0.0, "DUT set-up time"=0.0} ("Initialize Resource Config - Ganging"), "Master resource name"=w202, "Slave resource names"=w201, "System configuration"=w200, "Voltage/current level"=w199, "Voltage/current level range"=w198, "Limit symmetry"=w197, "Voltage/current limit range"=w196, "Voltage/current limit low"=w195, "Voltage/current limit high"=w194, "Output function"=w193, "Sense"=w192, "Transient response"=w191, "Voltage/current gain bandwith"=w190, "Voltage/current compensation frequency"=w189, "Voltage/current pole-zero ratio"=w188, "DUT set-up time"=1.0) -> (w209:T8)
        n48 = call "Initialize Resource Config-Ganging.vi"("error in"=w205, "Initialize Resource Config - Ganging"=w209) -> ("error out"=w187:errorcluster, "Ganged Session Out"=w208:T4)  [unwired: 8 in]
        n49 = Bundle By Name(cluster=w204, "Load Ganged Session Out"=w208) -> (w203:T3)
      }
      frame "SweepSource" {
        # "Get the sweep points for source"
        n50 = Unbundle By Name(w219) -> ("Source sweep scale"=w218:string, "Power ON V/I Source start level"=w217:dbl, "Source stop level"=w216:dbl, "Source sweep points/points per decade"=w215:i32)
        n51 = call "Calculate Sweep Values.vi"("Sweep type"=w218, "error in"=w220, "Points"=w215, "Stop level"=w216, "Start level"=w217) -> ("error out"=w210:errorcluster, "Sweep points"=w212:i32, "Sweep values"=w213:dbl[])  [unwired: 4 in]
        n52 = Bundle By Name(cluster=w214, "Source sweep values"=w213, "Source sweep points"=w212, "Measurement Results.Source sweep points"=w212) -> (w211:T3)
      }
      frame "SweepLoad" {
        # "Get the sweep points for load"
        n53 = Unbundle By Name(w230) -> ("Load sweep scale"=w229:string, "Load start level"=w228:dbl, "Load stop level"=w227:dbl, "Load sweep points/points per decade"=w226:i32)
        n54 = call "Calculate Sweep Values.vi"("Sweep type"=w229, "error in"=w231, "Points"=w226, "Stop level"=w227, "Start level"=w228) -> ("error out"=w222:errorcluster, "Sweep points"=w223:i32, "Sweep values"=w221:dbl[])  [unwired: 4 in]
        n55 = Bundle By Name(cluster=w225, "Load sweep values"=w221, "Load sweep points"=w223, "Measurement Results.Load sweep points"=w223) -> (w224:T3)
      }
      frame "ConfigureSourceToSequenceSingle" {
        # "Configure source to single sequence"
        n56 = Unbundle By Name(w248) -> ("Source channel name"=w244:string, "Source session out"=w245:refnum<k15>, "Source sweep values"=w246:dbl[], "Load sweep points"=w243:i32)
        n57 = Unbundle By Name(w247) -> ("Power ON/Source output function"=w242:i32, "Source transient response"=w241:i32, "Source voltage/current gain bandwidth"=w240:dbl, "Source voltage/current compensation frequency"=w239:dbl, "Source voltage/current pole-zero ratio"=w238:dbl, "Source aperture time"=w237:dbl, "Source source delay"=w236:dbl)
        n58 = Bundle By Name(cluster=T9 {"Source channel name"="", "Source out"="", "Source sweep values"=[], "Load sweep points"=0, "Source output function"=1006, "Source transient response"=1038, "Source voltage/current gain bandwidth"=0.0, "Source voltage/current compensation frequency"=0.0, "Source voltage/current pole-zero ratio"=0.0, "Source aperture time"=0.0, "Source source delay"=0.0} ("Source to seq config - Single"), "Source channel name"=w244, "Source out"=w245, "Source sweep values"=w246, "Load sweep points"=w243, "Source output function"=w242, "Source transient response"=w241, "Source voltage/current gain bandwidth"=w240, "Source voltage/current compensation frequency"=w239, "Source voltage/current pole-zero ratio"=w238, "Source aperture time"=w237, "Source source delay"=w236) -> (w232:T9)
        n59 = call "Configure Source to Sequence-Single.vi"("error in"=w235, "Source to seq config - Single"=w232) -> ("error out"=w234:errorcluster, "Source channel name"=w250:string, "instrument handle out"=w251:refnum<k15>)  [unwired: 7 in]
        n60 = Bundle By Name(cluster=w248, "Source session out"=w251, "Source channel name"=w250) -> (w249:T3)
      }
      frame "ConfigureSourceToSequenceGanged" {
        # "Configure source to ganged"
        n61 = Unbundle By Name(w266) -> ("Source Ganged Session Out"=w258:T4, "Source sweep values"=w257:dbl[], "Load sweep points"=w256:i32)
        n62 = Unbundle By Name(w267) -> ("Power ON/Source output function"=w259:i32, "Source transient response"=w260:i32, "Source voltage/current gain bandwidth"=w261:dbl, "Source voltage/current compensation frequency"=w262:dbl, "Source voltage/current pole-zero ratio"=w263:dbl, "Source aperture time"=w264:dbl, "Source source delay"=w265:dbl)
        n63 = Bundle By Name(cluster=T10 {"Source Ganged Session Out"={"Ganged Config"=enum."Series", "Session List"=[], "Session Mode"=[], "Channel"=[]}, "Source sweep values"=[], "Load sweep points"=0, "Source output function"=1006, "Source transient response"=1038, "Source voltage/current gain bandwidth"=0.0, "Source voltage/current compensation frequency"=0.0, "Source voltage/current pole-zero ratio"=0.0, "Source aperture time"=0.0, "Source source delay"=0.0} ("Source to seq config - Ganging"), "Source Ganged Session Out"=w258, "Source sweep values"=w257, "Load sweep points"=w256, "Source output function"=w259, "Source transient response"=w260, "Source voltage/current gain bandwidth"=w261, "Source voltage/current compensation frequency"=w262, "Source voltage/current pole-zero ratio"=w263, "Source aperture time"=w264, "Source source delay"=w265) -> (w252:T10)
        n64 = call "Configure Source to Sequence-Ganging.vi"("error in"=w255, "Source to seq config - Ganging"=w252) -> ("error out"=w254:errorcluster, "Ganged Session Out"=w268:T4)  [unwired: 8 in]
        n65 = Bundle By Name(cluster=w266, "Source Ganged Session Out"=w268) -> (w269:T3)
      }
      frame "ConfigureLoadToSequenceSingle" {
        # "Configure load to single"
        n66 = Unbundle By Name(w289) -> ("Load channel name"=w287:string, "Load session out"=w286:refnum<k15>, "Load sweep values"=w285:dbl[], "Source sweep points"=w284:i32)
        n67 = Unbundle By Name(w288) -> ("Load output function"=w283:i32, "Load transient response"=w282:i32, "Load voltage/current gain bandwidth"=w281:dbl, "Load voltage/current compensation frequency"=w280:dbl, "Load voltage/current pole-zero ratio"=w279:dbl, "Load aperture time"=w278:dbl, "Load source delay"=w277:dbl, "Load measure trigger"=w276:string, "Load source trigger"=w275:string)
        n68 = Bundle By Name(cluster=T11 {"Load channel name"="", "Load out"="", "Load sweep values"=[], "Source sweep points"=0, "Load output function"=1007, "Load transient response"=1038, "Load voltage/current gain bandwidth"=0.0, "Load voltage/current compensation frequency"=0.0, "Load voltage/current pole-zero ratio"=0.0, "Load aperture time"=0.0, "Load source delay"=0.0, "Load measure trigger"="", "Load source trigger"=""} ("Load to seq config - Single"), "Load channel name"=w287, "Load out"=w286, "Load sweep values"=w285, "Source sweep points"=w284, "Load output function"=w283, "Load transient response"=w282, "Load voltage/current gain bandwidth"=w281, "Load voltage/current compensation frequency"=w280, "Load voltage/current pole-zero ratio"=w279, "Load aperture time"=w278, "Load source delay"=w277, "Load measure trigger"=w276, "Load source trigger"=w275) -> (w271:T11)
        n69 = call "Configure Load to Sequence-Single.vi"("error in"=w274, "Load to seq config - Single"=w271) -> ("error out"=w273:errorcluster, "Load channel Name"=w270:string, "instrument handle out"=w290:refnum<k15>)  [unwired: 7 in]
        n70 = Bundle By Name(cluster=w289, "Load session out"=w290, "Load channel name"=w270) -> (w291:T3)
      }
      frame "ConfigureLoadToSequenceGanged" {
        # "Configure load to ganged"
        n71 = Unbundle By Name(w309) -> ("Load Ganged Session Out"=w307:T4, "Load sweep values"=w306:dbl[], "Source sweep points"=w305:i32)
        n72 = Unbundle By Name(w308) -> ("Load output function"=w304:i32, "Load transient response"=w303:i32, "Load voltage/current gain bandwidth"=w302:dbl, "Load voltage/current compensation frequency"=w301:dbl, "Load voltage/current pole-zero ratio"=w300:dbl, "Load aperture time"=w299:dbl, "Load source delay"=w298:dbl, "Load measure trigger"=w297:string, "Load source trigger"=w296:string)
        n73 = Bundle By Name(cluster=T12 {"Load Ganged Session Out"={"Ganged Config"=enum."Series", "Session List"=[], "Session Mode"=[], "Channel"=[]}, "Load sweep values"=[], "Source sweep points"=0, "Load output function"=1007, "Load transient response"=1038, "Load voltage/current gain bandwidth"=0.0, "Load voltage/current compensation frequency"=0.0, "Load voltage/current pole-zero ratio"=0.0, "Load aperture time"=0.0, "Load source delay"=0.0, "Load measure trigger"="", "Load source trigger"=""} ("Load to seq config - Ganging"), "Load Ganged Session Out"=w307, "Load sweep values"=w306, "Source sweep points"=w305, "Load output function"=w304, "Load transient response"=w303, "Load voltage/current gain bandwidth"=w302, "Load voltage/current compensation frequency"=w301, "Load voltage/current pole-zero ratio"=w300, "Load aperture time"=w299, "Load source delay"=w298, "Load measure trigger"=w297, "Load source trigger"=w296) -> (w292:T12)
        n74 = call "Configure Load to Sequence-Ganging.vi"("error in"=w295, "Load to seq config - Ganging"=w292) -> ("error out"=w294:errorcluster, "Ganged Session Out"=w310:T4)  [unwired: 8 in]
        n75 = Bundle By Name(cluster=w309, "Load Ganged Session Out"=w310) -> (w311:T3)
      }
      frame "StartAndWaitforEvent" {
        w326 = T14 1033 items=["Source Complete Event"=1030, "Measure Complete Event"=1031, "Sequence Iteration Complete Event"=1032, "Sequence Engine Done Event"=1033, "Pulse Complete Event"=1051, "Ready For Pulse Trigger Event"=1052] ("event")
        # "Wait for event"
        n76 = Unbundle By Name(w325) -> ("Source Ganged Session Out"=w334:T4, "Load Ganged Session Out"=w333:T4, "Source session out"=w332:refnum<k15>, "Load session out"=w331:refnum<k15>, "Source channel name"=w330:string, "Load channel name"=w329:string, "Load Source ON/OFF"=w312:T19, "Load ganged/single"=w328:bool, "Source ganged/single"=w327:bool)
        n77 = Bundle By Name(cluster=T13 {"Source Ganged Session Out"={"Ganged Config"=enum."Series", "Session List"=[], "Session Mode"=[], "Channel"=[]}, "Load Ganged Session Out"={"Ganged Config"=enum."Series", "Session List"=[], "Session Mode"=[], "Channel"=[]}, "Source session out"="", "Load session out"="", "event"=1030, "Source channel name"="", "Load channel name"="", "Load Source ON/OFF"=enum."SOURCE AND LOAD OFF", "Load ganged/single"=FALSE, "Source ganged/single"=FALSE} ("Start and wait event config"), "Source Ganged Session Out"=w334, "Load Ganged Session Out"=w333, "Source session out"=w332, "Load session out"=w331, "Source channel name"=w330, "Load channel name"=w329, "Load Source ON/OFF"=w312, "Load ganged/single"=w328, "Source ganged/single"=w327, "event"=w326) -> (w313:T13)
        n78 = call "Start and Wait for Event.vi"("error in"=w317, "Start and wait event config"=w313) -> ("error out"=w316:errorcluster, "Start and wait event result"=w315:T13)  [unwired: 7 in]
        n79 = Unbundle By Name(w315) -> ("Source Ganged Session Out"=w323:T4, "Load Ganged Session Out"=w322:T4, "Source session out"=w321:refnum<k15>, "Load session out"=w320:refnum<k15>, "Source channel name"=w319:string, "Load channel name"=w318:string)
        n80 = Bundle By Name(cluster=w325, "Source Ganged Session Out"=w323, "Load Ganged Session Out"=w322, "Source session out"=w321, "Load session out"=w320, "Source channel name"=w319, "Load channel name"=w318) -> (w324:T3)
      }
      frame "PerformMeasurement" {
        # "Fetch Measurement"
        n81 = Unbundle By Name(w355) -> ("Load Source ON/OFF"=w354:T19, "Source Ganged Session Out"=w353:T4, "Load Ganged Session Out"=w352:T4, "Source sweep values"=w351:dbl[], "Source sweep points"=w350:i32, "Load sweep values"=w349:dbl[], "Load sweep points"=w348:i32, "Measurement Results"=w347:T1, "Load ganged/single"=w346:bool, "Source ganged/single"=w345:bool, "Source channel name"=w344:string, "Load channel name"=w343:string, "Source session out"=w342:refnum<k15>, "Load session out"=w341:refnum<k15>)
        n82 = Unbundle By Name(w336) -> ("Measurement timeout"=w335:dbl)
        n83 = Bundle By Name(cluster=T15 {"Source Ganged Session Out"={"Ganged Config"=enum."Series", "Session List"=[], "Session Mode"=[], "Channel"=[]}, "Load Ganged Session Out"={"Ganged Config"=enum."Series", "Session List"=[], "Session Mode"=[], "Channel"=[]}, "Source sweep values"=[], "Source sweep points"=0, "Load sweep values"=[], "Load sweep points"=0, "Measurement Results"={"Status"="", "Source sweep points"=0, "Load sweep points"=0, "Source sweep values"=[], "Load sweep values"=[], "Source voltages"=[], "Source currents"=[], "Load voltages"=[], "Load currents"=[], "Eload status"=""}, "Load ganged/single"=FALSE, "Source ganged/single"=FALSE, "Source channel name"="", "Load channel name"="", "Source session out"="", "Load session out"="", "Load Source ON/OFF"=enum."SOURCE AND LOAD OFF", "Measurement timeout"=10.0} ("Sweep fetch measurement control"), "Load Source ON/OFF"=w354, "Source Ganged Session Out"=w353, "Load Ganged Session Out"=w352, "Source sweep values"=w351, "Source sweep points"=w350, "Load sweep values"=w349, "Load sweep points"=w348, "Measurement Results"=w347, "Load ganged/single"=w346, "Source ganged/single"=w345, "Source channel name"=w344, "Load channel name"=w343, "Source session out"=w342, "Load session out"=w341, "Measurement timeout"=w335) -> (w337:T15)
        n84 = call "Fetch Measurement-Sweep.vi"("error in (no error)"=w340, "Measure Call Context in"=w338, "Sweep fetch measurement control"=w337) -> ("error out"=w359:errorcluster, "Sweep fetch measurement"=w339:T15)  [unwired: 7 in]
        n85 = Unbundle By Name(w339) -> ("Measurement Results"=w356:T1)
        n86 = Bundle By Name(cluster=w355, "Measurement Results"=w356) -> (w357:T3)
      }
      frame "AbortAndCloseSession" {
        # "Abort and close session"
        n87 = Unbundle By Name(w362) -> ("Load Source ON/OFF"=w367:T19, "Source ganged/single"=w365:bool, "Load ganged/single"=w366:bool)
        n88 = case shown="\"SOURCE AND LOAD ON\"" w367 {
          tunnel: w365 -> [_ w375 _ w425]
          tunnel: w362 -> [_ w374 w398 w422]
          tunnel: w366 -> [_ _ w396 w426]
          tunnel: [w370 w372 w397 w415] -> w363
          tunnel: w360 -> [w370 w373 w399 w421]
          tunnel: ["" ("t") "" w389 w414] -> w361
          tunnel: w362 -> [_ _ w390 w413]
          frame Default {
          }
          frame "SOURCE ON" {
            # "Source enable"
            n89 = case shown="True" w375 {
              tunnel: w374 -> [w381 w388]
              tunnel: [w376 w384] -> w372
              tunnel: w373 -> [w380 w385]
              frame False {
                # "Ganged channel abort"
                n90 = Unbundle By Name(w381) -> ("Source Ganged Session Out"=w377:T4)
                n91 = Bundle By Name(cluster=T16 {"Ganged Session in"={"Ganged Config"=enum."Series", "Session List"=[], "Session Mode"=[], "Channel"=[]}} ("Ganged Session Out"), "Ganged Session in"=w377) -> (w378:T16)
                n92 = call "Abort Single Point-Ganging.vi"("error in"=w380, "Ganged Session In"=w378) -> ("error out"=w376:errorcluster)  [unwired: 9 in]
              }
              frame True {
                # "Single channel abort"
                n93 = Unbundle By Name(w388) -> ("Source session out"=w387:refnum<k15>, "Source channel name"=w386:string)
                n94 = Bundle By Name(cluster=T17 {"Resource out"="", "Resource channel name"=""} ("Abort Single Point - Single"), "Resource out"=w387, "Resource channel name"=w386) -> (w382:T17)
                n95 = call "Abort Single Point-Single.vi"("error in"=w385, "Abort Single Point - Single"=w382) -> ("error out"=w384:errorcluster)  [unwired: 9 in]
              }
            }
          }
          frame "LOAD ON" {
            (unwired) i16 3 ("width (-)")
            # "Load enable"
            n96 = case shown="True" w396 {
              tunnel: w398 -> [w405 w412]
              tunnel: [w403 w408] -> w397
              tunnel: w399 -> [w404 w409]
              frame False {
                # "Ganged channel abort"
                n97 = Unbundle By Name(w405) -> ("Source Ganged Session Out"=w400:T4)
                n98 = Bundle By Name(cluster=T16 {"Ganged Session in"={"Ganged Config"=enum."Series", "Session List"=[], "Session Mode"=[], "Channel"=[]}} ("Ganged Session Out"), "Ganged Session in"=w400) -> (w401:T16)
                n99 = call "Abort Single Point-Ganging.vi"("error in"=w404, "Ganged Session In"=w401) -> ("error out"=w403:errorcluster)  [unwired: 9 in]
              }
              frame True {
                # "Single channel abort"
                n100 = Unbundle By Name(w412) -> ("Load session out"=w411:refnum<k15>, "Load channel name"=w410:string)
                n101 = Bundle By Name(cluster=T17 {"Resource out"="", "Resource channel name"=""} ("Abort Single Point - Single"), "Resource out"=w411, "Resource channel name"=w410) -> (w406:T17)
                n102 = call "Abort Single Point-Single.vi"("error in"=w409, "Abort Single Point - Single"=w406) -> ("error out"=w408:errorcluster)  [unwired: 9 in]
              }
            }
            n103 = Unbundle By Name(w390) -> ("Number of Eload used"=w395:i32)
            n104 = Number To Decimal String(number=w395) -> (decimal integer string=w394:string)  [unwired: 1 in]
            n105 = Concatenate Strings("NO. OF E-LOAD USED: ", w394) -> (w393:string)
            n106 = Select(t="", s=w397, f=w393) -> (s? t:f=w389:string)
          }
          frame "SOURCE AND LOAD ON" {
            # "Source enable and load enable"
            n107 = Build Array(w425, w426) -> (w424:bool[])
            n108 = Boolean Array To Number(Boolean array=w424) -> (number=w423:u32)
            n109 = case shown="3" w423 {
              tunnel: w422 -> [w436 w447 w458 w468]
              tunnel: [w430 w438 w450 w459] -> w415
              tunnel: w421 -> [w429 w439 w453 w461]
              frame 0, Default {
                # "Source and load ganged abort"
                n110 = Unbundle By Name(w436) -> ("Source Ganged Session Out"=w434:T4, "Load Ganged Session Out"=w435:T4)
                n111 = Bundle By Name(cluster=T16 {"Ganged Session in"={"Ganged Config"=enum."Series", "Session List"=[], "Session Mode"=[], "Channel"=[]}} ("Ganged Session In"), "Ganged Session in"=w434) -> (w431:T16)
                n112 = Bundle By Name(cluster=T16 {"Ganged Session in"={"Ganged Config"=enum."Series", "Session List"=[], "Session Mode"=[], "Channel"=[]}} ("Ganged Session In"), "Ganged Session in"=w435) -> (w427:T16)
                n113 = call "Abort Single Point-Ganging.vi"("error in"=w429, "Ganged Session In"=w427) -> ("error out"=w428:errorcluster)  [unwired: 9 in]
                n114 = call "Abort Single Point-Ganging.vi"("error in"=w428, "Ganged Session In"=w431) -> ("error out"=w430:errorcluster)  [unwired: 9 in]
              }
              frame 1 {
                # "Source single load ganged abort"
                n115 = Unbundle By Name(w447) -> ("Source session out"=w445:refnum<k15>, "Source channel name"=w444:string, "Load Ganged Session Out"=w446:T4)
                n116 = Bundle By Name(cluster=T17 {"Resource out"="", "Resource channel name"=""} ("Abort Single Point - Single"), "Resource out"=w445, "Resource channel name"=w444) -> (w441:T17)
                n117 = Bundle By Name(cluster=T16 {"Ganged Session in"={"Ganged Config"=enum."Series", "Session List"=[], "Session Mode"=[], "Channel"=[]}} ("Ganged Session In"), "Ganged Session in"=w446) -> (w437:T16)
                n118 = call "Abort Single Point-Ganging.vi"("error in"=w439, "Ganged Session In"=w437) -> ("error out"=w440:errorcluster)  [unwired: 9 in]
                n119 = call "Abort Single Point-Single.vi"("error in"=w440, "Abort Single Point - Single"=w441) -> ("error out"=w438:errorcluster)  [unwired: 9 in]
              }
              frame 2 {
                # "Source ganged load single abort"
                n120 = Unbundle By Name(w458) -> ("Source Ganged Session Out"=w455:T4, "Load session out"=w457:refnum<k15>, "Load channel name"=w456:string)
                n121 = Bundle By Name(cluster=T17 {"Resource out"="", "Resource channel name"=""} ("Abort Single Point - Single"), "Resource out"=w457, "Resource channel name"=w456) -> (w448:T17)
                n122 = Bundle By Name(cluster=T16 {"Ganged Session in"={"Ganged Config"=enum."Series", "Session List"=[], "Session Mode"=[], "Channel"=[]}} ("Ganged Session In"), "Ganged Session in"=w455) -> (w451:T16)
                n123 = call "Abort Single Point-Single.vi"("error in"=w453, "Abort Single Point - Single"=w448) -> ("error out"=w449:errorcluster)  [unwired: 9 in]
                n124 = call "Abort Single Point-Ganging.vi"("error in"=w449, "Ganged Session In"=w451) -> ("error out"=w450:errorcluster)  [unwired: 9 in]
              }
              frame 3 {
                # "Source and load single abort"
                n125 = Unbundle By Name(w468) -> ("Source session out"=w466:refnum<k15>, "Source channel name"=w467:string, "Load session out"=w470:refnum<k15>, "Load channel name"=w469:string)
                n126 = Bundle By Name(cluster=T17 {"Resource out"="", "Resource channel name"=""} ("Abort Single Point - Single"), "Resource out"=w466, "Resource channel name"=w467) -> (w463:T17)
                n127 = Bundle By Name(cluster=T17 {"Resource out"="", "Resource channel name"=""} ("Abort Single Point - Single"), "Resource out"=w470, "Resource channel name"=w469) -> (w462:T17)
                n128 = call "Abort Single Point-Single.vi"("error in"=w461, "Abort Single Point - Single"=w462) -> ("error out"=w460:errorcluster)  [unwired: 9 in]
                n129 = call "Abort Single Point-Single.vi"("error in"=w460, "Abort Single Point - Single"=w463) -> ("error out"=w459:errorcluster)  [unwired: 9 in]
              }
            }
            n130 = Unbundle By Name(w413) -> ("Number of Eload used"=w420:i32)
            n131 = Number To Decimal String(number=w420) -> (decimal integer string=w419:string)  [unwired: 1 in]
            n132 = Concatenate Strings("NO. OF E-LOAD USED: ", w419) -> (w418:string)
            n133 = Select(t="", s=w415, f=w418) -> (s? t:f=w414:string)
          }
        }
        n134 = Bundle By Name(cluster=w362, "Measurement Results.Eload status"=w361) -> (w364:T3)
      }
      frame "Exit", Default {
        n135 = case shown="No Error" w473 {
          selector: w473 -> [w478 w479]
          tunnel: [w477 w479] -> w472
          tunnel: w471 -> [w476 _]
          frame No Error {
            # "Release the queue"
            n136 = Release Queue(queue=w476, error in (no error)=w478) -> (error out=w477:errorcluster)  [unwired: 1 in, 2 out]
          }
          frame Error {
          }
        }
      }
    }
  }
  "error out" <- w17
  "Measure Call Context out" <- w15
  n137 = Unbundle By Name(w2) -> ("Measurement Results"=→"Measurement Results":T1)
